vi "upload_to_s3.vi"(8 "error in":errorcluster, 9 "timeout per chunk (ms)":i32=300000, 10 "File":path, 11 "Nominal Client in":refnum<class "Nominal Client.lvclass">) -> (0 "error out":errorcluster, 2 "source":refnum<class "s3.lvclass">, 3 "Nominal Client out":refnum<class "Nominal Client.lvclass">)   [LabVIEW 2020, in "Nominal Client.lvclass"]
doc: "Uploads a file to Nominal by taking the file path as input and automatically selecting the appropriate upload technique based on the file size. Small files are uploaded in a single operation, while large files are uploaded using a multipart strategy for efficiency and reliability."
uses:
  Nominal Client.lvclass
  datasources/s3/s3.lvclass
  Nominal Client.lvclass/Nominal Client.ctl
  datasources/source/source.lvclass
  datasources/source/create_s3.vi
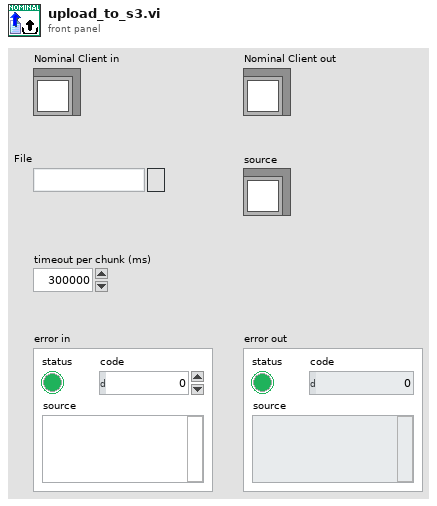
[diagram p1: front panel]
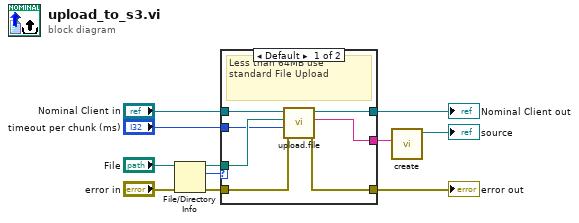
[diagram p0: block diagram]
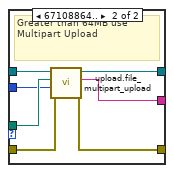
[diagram p2: hidden frame]
diagram:
  n1 = File/Directory Info(path="File", error in="error in") -> (path out=w8:path, size=w10:i64, error out=w5:errorcluster)  [unwired: 4 out]
  n2 = case shown="Default" w10 {
    tunnel: w8 -> [w18 w22]
    tunnel: "Nominal Client in" -> [w17 w25]
    tunnel: [w16 w24] -> w6
    tunnel: w5 -> [w15 w21]
    tunnel: [w14 w20] -> w4
    tunnel: [w13 w23] -> w3
    tunnel: "timeout per chunk (ms)" -> [w12 w19]
    frame Default {
      # "Less than 64MB use standard File Upload"
      n3 = call "upload.file.vi"("error in"=w15, "timeout (ms)"=w12, "File"=w18, "Nominal Client in"=w17) -> ("error out"=w14:errorcluster, "Path to S3 File"=w13:string, "Nominal Client out"=w16:refnum<class "Nominal Client.lvclass">)  [unwired: 5 in]
    }
    frame 67108864.. {
      # "Greater than 64MB use Multipart Upload"
      n4 = call "upload.file_multipart_upload.vi"("error in"=w21, "timeout per chunk (ms)"=w19, "File Path"=w22, "Nominal Client in"=w25) -> ("error out"=w20:errorcluster, "S3 Path to File"=w23:string, "Nominal Client out"=w24:refnum<class "Nominal Client.lvclass">)  [unwired: 5 in]
    }
  }
  "Nominal Client out" <- w6
  "error out" <- w4
  n5 = call-poly "create.vi"("Path"=w3) -> ("source"=→"source":refnum<class "s3.lvclass">)  [unwired: 10 in]
